vi "Untitled 5 (SubVI).vi"(0 "UI in":refnum<class "UI Actor.lvclass">, 1 "Last Ack":refnum<class "Last Ack.lvclass">, 5 "error in (no error)":errorcluster) -> (14 "UI out":refnum<class "UI Actor.lvclass">, 19 "error out":errorcluster)   [LabVIEW 2014, in "Device Test.lvlib" / "UI Actor.lvclass"]
uses:
  UI Actor.lvclass
  <vilib>/ActorFramework/LastAck/Last Ack.lvclass
  UI Actor.lvclass/UI Actor.ctl
  <vilib>/ActorFramework/Actor/Actor.lvclass/Actor.ctl
  <vilib>/ActorFramework/Message Enqueuer/Message Enqueuer.lvclass/Message Enqueuer.ctl
  <vilib>/ActorFramework/Message Enqueuer/Init from Existing Queue.vi
  <vilib>/ActorFramework/Message Enqueuer/Enqueue.vi
  <vilib>/ActorFramework/Message Priority Queue/Priority Enqueue.vi
  <vilib>/ActorFramework/Message Enqueuer/Message Enqueuer.lvclass
  <vilib>/ActorFramework/Stop Msg/Stop Msg.lvclass
  <vilib>/ActorFramework/Actor/Actor.lvclass
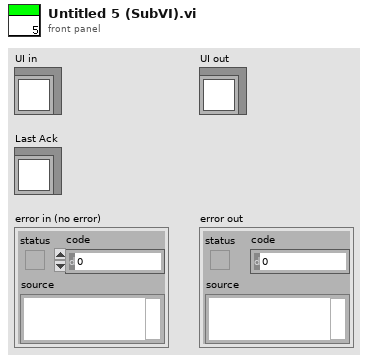
[diagram p1: front panel]
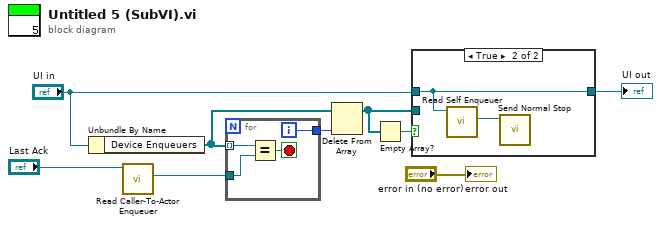
[diagram p0: block diagram]
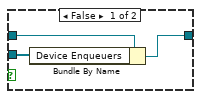
[diagram p2: hidden frame]
diagram:
  n1 = Unbundle By Name("UI in") -> ("Device Enqueuers"=w4:refnum<class "Message Enqueuer.lvclass">[])
  n2 = call <vilib>:"Read Caller-To-Actor Enqueuer.vi"("Last Ack"="Last Ack") -> ("Caller-to-Actor Enqueuer"=w3:refnum<class "Message Enqueuer.lvclass">)  [unwired: 10 in]
  n3 = for {
    tunnel: w4 -> [w13] mode=indexing
    tunnel: w3 -> [w12]
    tunnel: [w10] -> w5
    i -> [w10]
    stop <- w11 stop-if-true
    n4 = Equal?(x=w13, y=w12) -> (x = y?=w11:bool)
  }
  n5 = Delete From Array(array=w4, index=w5) -> (array with subset deleted=w6:refnum<class "Message Enqueuer.lvclass">[])  [unwired: 1 in, 1 out]
  n6 = Empty Array?(array=w6) -> (empty?=w9:bool)
  n7 = case shown="True" w9 {
    tunnel: w6 -> [w16 _]
    tunnel: [w15 w18] -> w7
    tunnel: "UI in" -> [w14 w18]
    frame False {
      n8 = Bundle By Name(cluster=w14, "Device Enqueuers"=w16) -> (w15:refnum<class "UI Actor.lvclass">)
    }
    frame True {
      n9 = call <vilib>:"Read Self Enqueuer.vi"("Actor"=w18) -> ("Self Enqueuer"=w17:refnum<class "Message Enqueuer.lvclass">)  [unwired: 10 in]
      n10 = call <vilib>:"Send Normal Stop.vi"("Message Enqueuer"=w17) -> ()  [unwired: 10 in, 1 out]
    }
  }
  "UI out" <- w7
  "error out" <- "error in (no error)"
